vi "random-competition.vi"() -> ()   [LabVIEW 2023]
panel:
  out "Winner B":bool
  out "Tie":bool
  out "Winner A":bool
  out "Random Number A":dbl
  out "Points B":i32
  out "Points A":i32
  out "Random Number B":dbl
  in  "Number of Iterations":i32
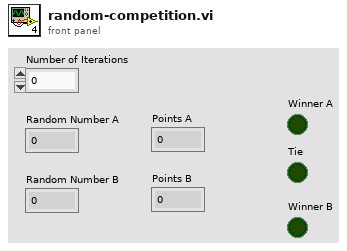
[diagram p1: front panel]
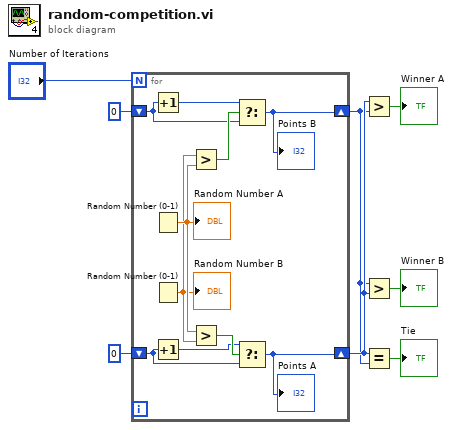
[diagram p0: block diagram]
diagram:
  n1 = for {
    N: "Number of Iterations" -> [_]
    shift-right: [w9] -> w3
    shift-left: 0 -> [w13]
    shift-right: [w10] -> w2
    shift-left: 0 -> [w16]
    n2 = Increment(x=w16) -> (x+1=w17:i32)
    n3 = Random Number (0-1)() -> (number: 0 to 1=w12:dbl)
    "Random Number A" <- w12
    n4 = Random Number (0-1)() -> (number: 0 to 1=w11:dbl)
    "Random Number B" <- w11
    n5 = Increment(x=w13) -> (x+1=w14:i32)
    n6 = Greater?(x=w11, y=w12) -> (0:w18:bool)
    n7 = Greater?(x=w12, y=w11) -> (0:w15:bool)
    n8 = Select(t=w17, s=w18, f=w16) -> (s? t:f=w10:i32)
    "Points B" <- w10
    n9 = Select(t=w14, s=w15, f=w13) -> (s? t:f=w9:i32)
    "Points A" <- w9
  }
  n10 = Greater?(x=w3, y=w2) -> (0:→"Winner A":bool)
  n11 = Greater?(x=w2, y=w3) -> (0:→"Winner B":bool)
  n12 = Equal?(x=w3, y=w2) -> (x = y?=→"Tie":bool)
